vi "bold_lines.vi"(8 "error in (no error)":errorcluster, 10 "Lines to bold":i32[](array[numeric]), 11 "String reference in":refnum<vi>) -> (0 "error out":errorcluster, 3 "String reference out":refnum<vi>)   [LabVIEW 2020]
panel:
  # "Inputs"
  # "Outputs"
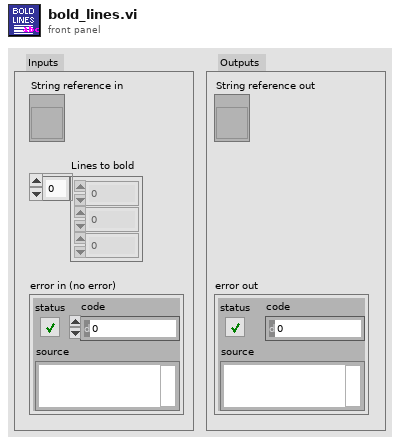
[diagram p1: front panel]
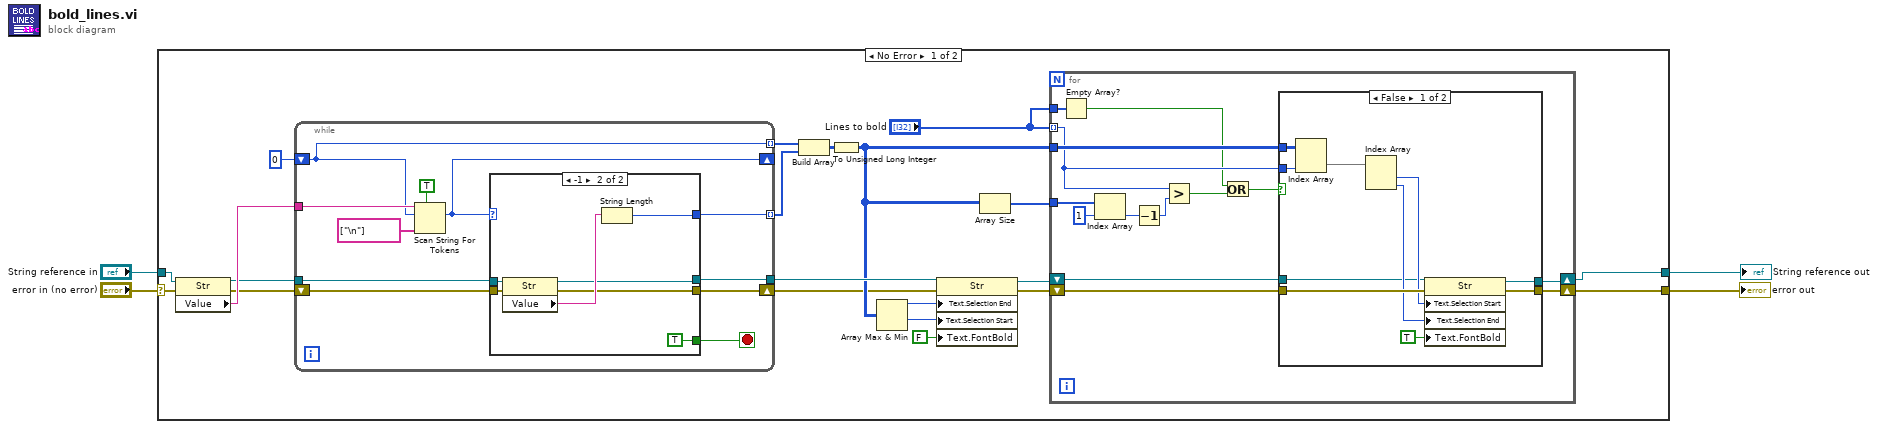
[diagram p0: block diagram]
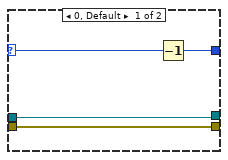
[diagram p3: hidden frame]
diagram:
  n1 = case shown="No Error" "error in (no error)" {
    selector: "error in (no error)" -> [w6 w74]
    tunnel: [w25 w75] -> w4
    tunnel: [w5 w74] -> w3
    tunnel: "String reference in" -> [w21 w75]
    frame No Error {
      n2 = property on="Property Node" class="Str"(reference=w21, error in=w6) -> (reference out=w23:refnum<vi>, error out=w22:errorcluster, "Value"=w24:string)
      n3 = while {
        shift-right: [w58] -> _
        shift-left: 0 ("offset past token") -> [w61]
        tunnel: w24 -> [w62]
        tunnel: [w61] -> w9 mode=indexing
        tunnel: [w60] -> w10 mode=indexing
        shift-right: [w54] -> w14
        shift-left: w22 -> [w55]
        tunnel: w23 -> [w53]
        tunnel: [w52] -> w19
        stop <- w56 stop-if-true
        n4 = Scan String For Tokens(5:TRUE ("allow empty tokens? (F)"), 6:string[] ["\n"] ("delimiters (\\s,\\t,\\r,\\n)"), 8:w61, 9:w62) -> (2:w58:i32)  [unwired: 2 in, 3 out]
        n5 = case shown="-1" w58 {
          selector: w58 -> [w65 _]
          tunnel: [w66 w72] -> w60
          tunnel: [_ TRUE] -> w56
          tunnel: w55 -> [w64 w70]
          tunnel: [w64 w69] -> w54
          tunnel: w53 -> [w63 w68]
          tunnel: [w63 w67] -> w52
          frame 0, Default {
            n6 = Decrement(x=w65) -> (x-1=w66:i32)
          }
          frame -1 {
            n7 = property on="Property Node" class="Str"(reference=w68, error in=w70) -> (reference out=w67:refnum<vi>, error out=w69:errorcluster, "Value"=w73:string)
            n8 = String Length(string=w73) -> (length=w72:i32)
          }
        }
      }
      n9 = Build Array(w9, w10) -> (w12:i32[][])
      n10 = To Unsigned Long Integer(number=w12) -> (unsigned 32bit integer=w17:u32[][])
      n11 = Array Max & Min(array=w17) -> (max value=w15:u32, min value=w16:u32)  [unwired: 2 out]
      n12 = property on="Property Node" class="Str"(reference=w19, error in=w14, "Text.Selection End"=w15, "Text.Selection Start"=w16, "Text.FontBold"=FALSE ("Text.Font:Bold")) -> (reference out=w20:refnum<vi>, error out=w13:errorcluster)
      n13 = Array Size(array=w17) -> (size(s)=w11:i32[])
      n14 = for {
        tunnel: "Lines to bold" -> [w38] mode=indexing
        tunnel: w17 -> [w39]
        tunnel: w11 -> [w37]
        shift-right: [w32] -> w5
        shift-left: w13 -> [w33]
        tunnel: "Lines to bold" -> [w29]
        shift-right: [w30] -> w25
        shift-left: w20 -> [w31]
        n15 = Empty Array?(array=w29) -> (empty?=w27:bool)
        n16 = Index Array(array=w37, index=1) -> (element=w36:i32)
        n17 = Decrement(x=w36) -> (x-1=w34:i32)
        n18 = Greater?(x=w38, y=w34) -> (0:w26:bool)
        n19 = Or(x=w27, y=w26) -> (x .or. y?=w28:bool)
        n20 = case shown="False" w28 {
          tunnel: w39 -> [w49 _]
          tunnel: w38 -> [w48 _]
          tunnel: w33 -> [w46 w51]
          tunnel: [w42 w51] -> w32
          tunnel: w31 -> [w41 w50]
          tunnel: [w40 w50] -> w30
          frame False {
            n21 = Index Array(array=w49, index (col)=w48) -> (element=w47:u32[])  [unwired: 1 in]
            n22 = Index Array(array=w47) -> (element #1=w45:u32, element #2=w44:u32)  [unwired: 2 in]
            n23 = property on="Property Node" class="Str"(reference=w41, error in=w46, "Text.Selection Start"=w45, "Text.Selection End"=w44, "Text.FontBold"=TRUE ("Text.Font:Bold")) -> (reference out=w40:refnum<vi>, error out=w42:errorcluster)
          }
          frame True {
          }
        }
      }
    }
    frame Error {
    }
  }
  "String reference out" <- w4
  "error out" <- w3
